vi "Remove Test.vi"(8 "error in (no error)":errorcluster, 10 "Unique ID":string, 11 "Test Executive in":refnum<class "Test Executive.lvclass">) -> (0 "error out":errorcluster, 2 "Orphaned Pointer IDs":string[](array[string]), 3 "Test Executive out":refnum<class "Test Executive.lvclass">)   [LabVIEW 2019, in "Test Executive.lvlib" / "Test Executive.lvclass"]
uses:
  <vilib>/gpm_packages/@cs/test-executive/Source/Test Executive/TestExecutive/Test Executive.lvclass
  <vilib>/gpm_packages/@cs/test-executive/Source/Test Executive/TestExecutive/Test Executive.lvclass/Test Executive.ctl
  958d93bb-7996-4a48-a796-a7764140f16b.vi
  69858890-0a2d-46f8-b109-284d73b69eac.vi
  <vilib>/gpm_packages/@cs/linked-list/Source/Linked List/ILinkedList/ILinked List.lvclass
  <vilib>/gpm_packages/@cs/linked-list/Source/Linked List/Linked List Ref/Linked List Ref.lvclass
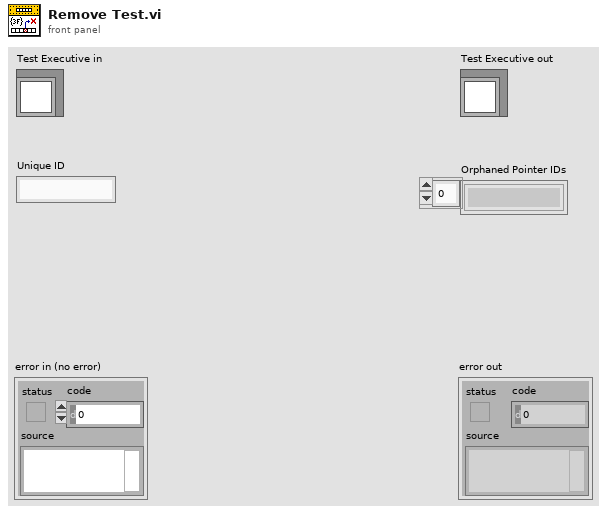
[diagram p1: front panel]
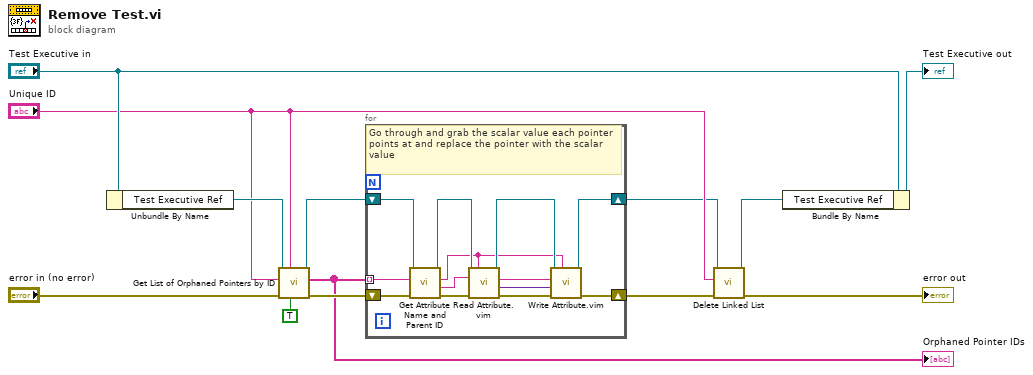
[diagram p0: block diagram]
diagram:
  n1 = Unbundle By Name("Test Executive in") -> ("Test Executive Ref"=w8:refnum<data-value>)
  n2 = call <vilib>:"Get List of Orphaned Pointers by ID.vi"("Recurse Up List"=TRUE, "Linked List ID"="Unique ID", "error in (no error)"="error in (no error)", "Removed Unique ID"="Unique ID", "Linked List Ref"=w8) -> ("error out"=w3:errorcluster, "Orphaned Pointer IDs"=w1:string[], "Linked List Ref out"=w5:refnum<data-value>)  [unwired: 4 in]
  "Orphaned Pointer IDs" <- w1
  n3 = for {
    shift-right: [w17] -> w4
    shift-left: w5 -> [w26]
    shift-right: [w19] -> w2
    shift-left: w3 -> [w24]
    tunnel: w1 -> [w22] mode=indexing
    # "Go through and grab the scalar value each pointer points at and replace the pointer with the scalar value"
    n4 = call <vilib>:"Get Attribute Name and Parent ID.vi"("error in (no error)"=w24, "Tag"=w22, "Linked List Ref"=w26) -> ("error out"=w23:errorcluster, "Attribute Name"=w21:string, "Linked List ID"=w16:string, "Linked List Ref out"=w25:refnum<data-value>)  [unwired: 5 in]
    n5 = call "Read Attribute.vim"("Linked List Ref"=w25, "Linked List ID"=w16, "Attribute Name"=w21, "error in (no error)"=w23) -> ("Linked List Ref out"=w18:refnum<data-value>, "Attribute Name out"=w15:string, "Attribute"=w14:variant, "error out"=w20:errorcluster)  [unwired: 6 in, 2 out]
    n6 = call "Write Attribute.vim"("Linked List ID"=w16, "error in (no error)"=w20, "Attribute"=w14, "Attribute Name"=w15, "Linked List Ref"=w18) -> ("error out"=w19:errorcluster, "Linked List Ref out"=w17:refnum<data-value>)  [unwired: 3 in, 2 out]
  }
  n7 = call <vilib>:"Delete Linked List.vi"("error in (no error)"=w2, "Linked List ID"="Unique ID", "Linked List Ref"=w4) -> ("error out"=→"error out":errorcluster, "Linked List Ref out"=w10:refnum<data-value>)  [unwired: 7 in]
  n8 = Bundle By Name(cluster="Test Executive in", "Test Executive Ref"=w10) -> (→"Test Executive out":refnum<class "Test Executive.lvclass">)
